vi "TWM Client Cmd Get Algorithm Info.vi"(7 "end of packet key":string="TWM:command:EndOfPacket", 8 "error in":errorcluster, 10 "algorithm id":string, 11 "handle":i32) -> (0 "error out":errorcluster, 2 "algorithm info":T1, 3 "handle out":i32)   [LabVIEW 2020, in "TWM Client.lvlib"]
doc: "Write Get algorithm info command packet to TWM server. Get answer."
uses:
  TWM Client.lvlib
  TWM Client Algorithm Info.ctl
  String.vi
  Get 1D String.vi
  <vilib>/Utility/error.llb/Error Cluster From Error Code.vi
  GetBoolean.vi
  GetString.vi
  <vilib>/ErrorRing/Error Ring.xnode
  infolib.lvlib
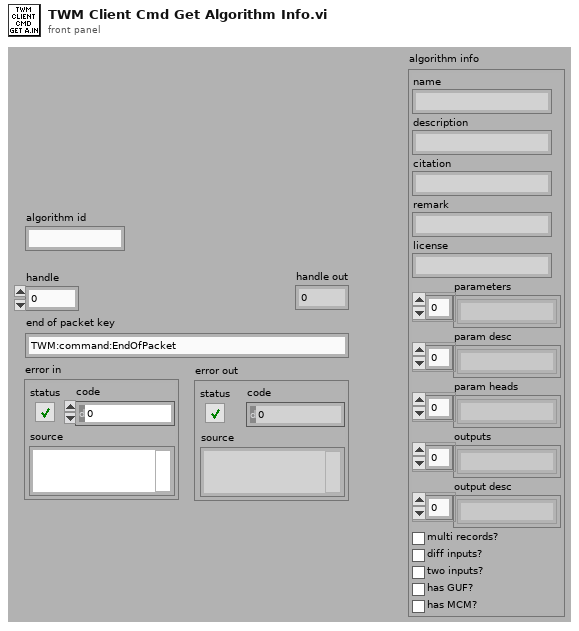
[diagram p1: front panel]
types:
  T1 = typedef "TWM Client.lvlib/TWM Client Algorithm Info.ctl" = cluster{"name":string, "description":string, "citation":string, "remark":string, "license":string, "parameters":string[], "param desc":string[], "param heads":string[], "outputs":string[], "output desc":string[], "multi records?":bool, "diff inputs?":bool, "two inputs?":bool, "has GUF?":bool, "has MCM?":bool}
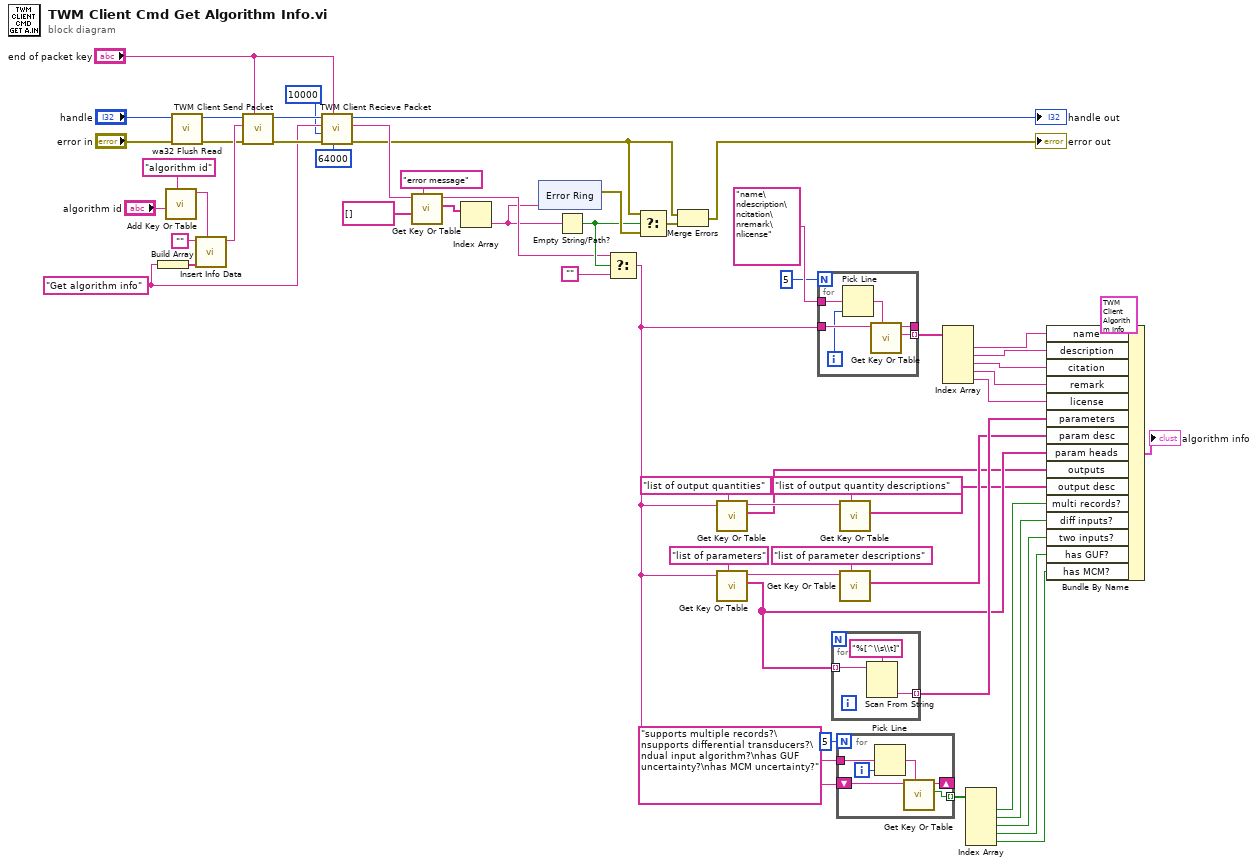
[diagram p0: block diagram]
diagram:
  w49 = "Get algorithm info" ("key string")
  n1 = Build Array(w49) -> (w50:string[])
  n2 = call-poly "Add Key Or Table.vi"("key description"="algorithm id", "string"="algorithm id") -> ("info data out"=w51:string)  [unwired: 8 in, 1 out]
  n3 = call "wa32 Flush Read.vi"("error in"="error in", "handle"="handle") -> ("error out"=w3:errorcluster, "handle out"=w2:i32)  [unwired: 7 in, 1 out]
  n4 = call "Insert Info Data.vi"("info data to insert"=w51, "sections"=w50, "info data"="") -> ("info data out"=w48:string)  [unwired: 7 in, 1 out]
  n5 = call "TWM Client Send Packet.vi"("end of packet key"="end of packet key", "error in"=w3, "command string"=w48, "handle"=w2) -> ("error out"=w58:errorcluster, "handle out"=w56:i32)  [unwired: 6 in]
  n6 = call "TWM Client Recieve Packet.vi"("max message length (1024)"=64000, "end of packet key"="end of packet key", "error in"=w58, "timeout [ms] (5000 ms)"=10000, "message header (empty)"=w49, "handle in"=w56) -> ("error out"=w43:errorcluster, "message data"=w53:string, "handle out"=→"handle out":i32)  [unwired: 3 in]
  n7 = call-poly "Get Key Or Table.vi"("key description"="error message", "string"=string[] [], "info data"=w53) -> ("value"=w44:string[], "info data out"=w40:string)  [unwired: 5 in, 2 out]
  n8 = Index Array(array=w44) -> (element=w6:string)  [unwired: 1 in]
  n9 = xnode "Error Ring"("parameter 0"=w6) -> ("error out"=w42:errorcluster)
  n10 = Empty String/Path?(string/path=w6) -> (empty?=w41:bool)
  n11 = Select(t=w40, s=w41, f="") -> (s? t:f=w5:string)
  n12 = Select(t=w43, s=w41, f=w42) -> (s? t:f=w47:errorcluster)
  n13 = Merge Errors(w43, w47) -> (→"error out":errorcluster)
  n14 = call-poly "Get Key Or Table.vi"("key description"="list of output quantities", "info data"=w5) -> ("value"=w17:string[], "info data out"=w19:string)  [unwired: 6 in, 2 out]
  n15 = call-poly "Get Key Or Table.vi"("key description"="list of parameters", "info data"=w5) -> ("value"=w23:string[], "info data out"=w34:string)  [unwired: 6 in, 2 out]
  n16 = for {
    N: 5 -> [_]
    tunnel: [w65] -> _
    tunnel: w5 -> [w64]
    tunnel: [w63] -> w32 mode=indexing
    tunnel: "name\ndescription\ncitation\nremark\nlicense" -> [w62]
    i -> [w60]
    n17 = Pick Line(multi-line string=w62, line index=w60) -> (output string=w61:string)  [unwired: 1 in]
    n18 = call-poly "Get Key Or Table.vi"("key description"=w61, "info data"=w64) -> ("value"=w63:string, "info data out"=w65:string)  [unwired: 6 in, 2 out]
  }
  n19 = for {
    tunnel: w23 -> [w68] mode=indexing
    tunnel: [w66] -> w25 mode=indexing
    n20 = Scan From String(format string="%[^\\s\\t]", input string=w68) -> (output 1=w66:string)  [unwired: 3 in, 3 out]
  }
  n21 = for {
    N: 5 -> [_]
    tunnel: "supports multiple records?\nsupports differential transducers?\ndual input algorithm?\nhas GUF uncertainty?\nhas MCM uncertainty?" -> [w72]
    shift-right: [w73] -> _
    shift-left: w5 -> [w74]
    tunnel: [w69] -> w14 mode=indexing
    i -> [w70]
    n22 = Pick Line(multi-line string=w72, line index=w70) -> (output string=w71:string)  [unwired: 1 in]
    n23 = call-poly "Get Key Or Table.vi"("key description"=w71, "info data"=w74) -> ("value"=w69:bool, "info data out"=w73:string)  [unwired: 6 in, 2 out]
  }
  n24 = call-poly "Get Key Or Table.vi"("key description"="list of output quantity descriptions", "info data"=w19) -> ("value"=w16:string[])  [unwired: 6 in, 3 out]
  n25 = call-poly "Get Key Or Table.vi"("key description"="list of parameter descriptions", "info data"=w34) -> ("value"=w24:string[])  [unwired: 6 in, 3 out]
  n26 = Index Array(array=w32) -> (element #1=w30:string, element #2=w29:string, element #3=w28:string, element #4=w27:string, element #5=w26:string)  [unwired: 5 in]
  n27 = Index Array(array=w14) -> (element #1=w13:bool, element #2=w12:bool, element #3=w11:bool, element #4=w9:bool, element #5=w8:bool)  [unwired: 5 in]
  n28 = Bundle By Name(cluster=T1 {"name"="", "description"="", "citation"="", "remark"="", "license"="", "parameters"=[], "param desc"=[], "param heads"=[], "outputs"=[], "output desc"=[], "multi records?"=FALSE, "diff inputs?"=FALSE, "two inputs?"=FALSE, "has GUF?"=FALSE, "has MCM?"=FALSE} ("alg info"), "name"=w30, "description"=w29, "citation"=w28, "remark"=w27, "license"=w26, "parameters"=w25, "param desc"=w24, "param heads"=w23, "outputs"=w17, "output desc"=w16, "multi records?"=w13, "diff inputs?"=w12, "two inputs?"=w11, "has GUF?"=w9, "has MCM?"=w8) -> (→"algorithm info":T1)
